vi "Untitled 2.vi"   [LabVIEW 2013]
types:
  T1 = typedef "cDAQ Chassis.ctl" = cluster{"ProductType":string, "DevSerialNum":u32, "Device Name":tag, "DevsInSlots":T2[]}
  T2 = typedef "IO Module Descriptor.ctl" = cluster{"CompactDAQ.SlotNum":u32, "Name":tag, "ProductType":string, "DevSerialNum":u32}
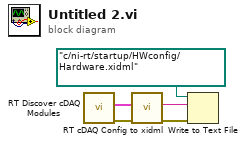
[diagram p0: block diagram]
diagram:
  n1 = call "RT Discover cDAQ Modules.vi"() -> ("Error Out"=w2:errorcluster, "Discovered Devices"=w5:T1[])  [unwired: 10 in]
  n2 = call "RT cDAQ Config to xidml.vi"("Error In"=w2, "Devices"=w5) -> ("Error Out"=w1:errorcluster, "xidml Out"=w4:string)  [unwired: 8 in]
  n3 = Write to Text File(file (use dialog)=path "c:/ni-rt/startup/HWconfig/Hardware.xidml" ("XML File Path"), text=w4, error in=w1) -> ()  [unwired: 1 in, 3 out]
